vi "Generate_WayPoints_ConstantDistance_Unidirection_DPS_and_CV_V2.vi"(11 "Input Cluster":T2={"Scan Rate (um/s)"=15.0, "X Start"=15.0, "X End"=15.0, "Y Start"=15.0, "Y End"=15.0, "Z Start"=15.0, "Moving Distance (um)"=1.0, "V"=15.0, "Z End"=15.0, "V2"=15.0, "Approach Rate (um/s)"=15.0, "V3"=15.0, "CV Rate (V/s)"=15.0, " V4"=15.0, "V1"=15.0, "Hold Time1 (ms)"=15, "Hold Time2 (ms)"=15, "Hold Time3 (ms)"=15, "Hold Time4 (ms)"=15, "Hold Time5 (ms)"=15, "Update Position Loop Wait Time (us)"=50000, " V5"=15.0, "Hold Time at each point (ms)"=2, "Backward rate (um/s)"=15.0, "Double potential step feedback? (T/F)"=TRUE, "Hold Time6 (ms)"=15, "Hold Time6 (ms) after move"=15, "From V5 to V,\npotential step (true) or\npotential sweep (false)"=TRUE}) -> (0 "output cluster":T1)   [LabVIEW 2023]
uses:
  TypeDefs/WayPointCluster.ctl
panel:
  in  "WayPointCluster":T1
  out "Y  P":dbl
  out "X  P":dbl
  out "HoppingDistanceX":dbl
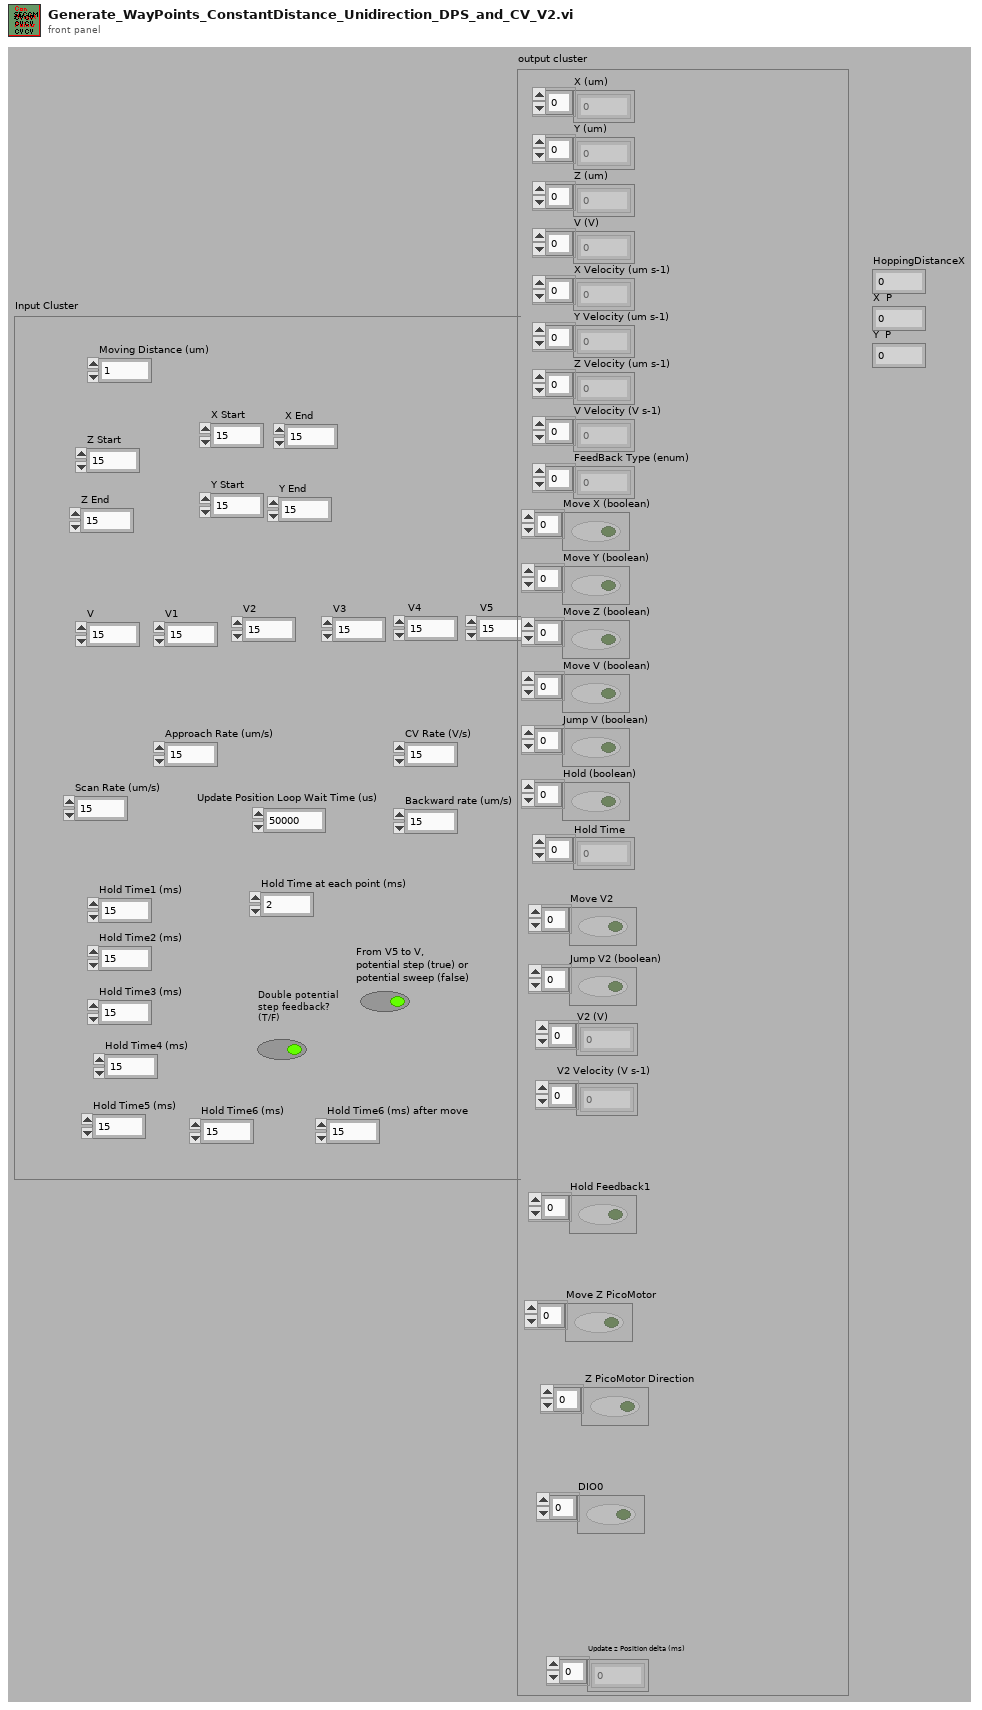
[diagram p1: front panel]
types:
  T1 = typedef "WayPointCluster.ctl" = cluster{"X (um)":dbl[], "Y (um)":dbl[], "Z (um)":dbl[], "V (V)":dbl[], "X Velocity (um s-1)":dbl[], "Y Velocity (um s-1)":dbl[], "Z Velocity (um s-1)":dbl[], "V Velocity (V s-1)":dbl[], "FeedBack Type (enum)":u16[], "Move X (boolean)":bool[], "Move Y (boolean)":bool[], "Move Z (boolean)":bool[], "Move V (boolean)":bool[], "Jump V (boolean)":bool[], "Hold (boolean)":bool[], "Hold Time":u32[], "V2 (V)":dbl[], "Move V2":bool[], "V2 Velocity (V s-1)":dbl[], "Jump V2 (boolean)":bool[], "Update z Position delta (ms)":i16[], "Hold Feedback1":bool[], "Move Z PicoMotor":bool[], " Z PicoMotor Direction":bool[], "DIO0":bool[]}
  T2 = cluster{"Scan Rate (um/s)":dbl, "X Start":dbl, "X End":dbl, "Y Start":dbl, "Y End":dbl, "Z Start":dbl, "Moving Distance (um)":dbl, "V":dbl, "Z End":dbl, "V2":dbl, "Approach Rate (um/s)":dbl, "V3":dbl, "CV Rate (V/s)":dbl, " V4":dbl, "V1":dbl, "Hold Time1 (ms)":i32, "Hold Time2 (ms)":i32, "Hold Time3 (ms)":i32, "Hold Time4 (ms)":i32, "Hold Time5 (ms)":i32, "Update Position Loop Wait Time (us)":u32, " V5":dbl, "Hold Time at each point (ms)":i32, "Backward rate (um/s)":dbl, "Double potential step feedback? (T/F)":bool, "Hold Time6 (ms)":i32, "Hold Time6 (ms) after move":i32, "From V5 to V,\npotential step (true) or\npotential sweep (false)":bool}
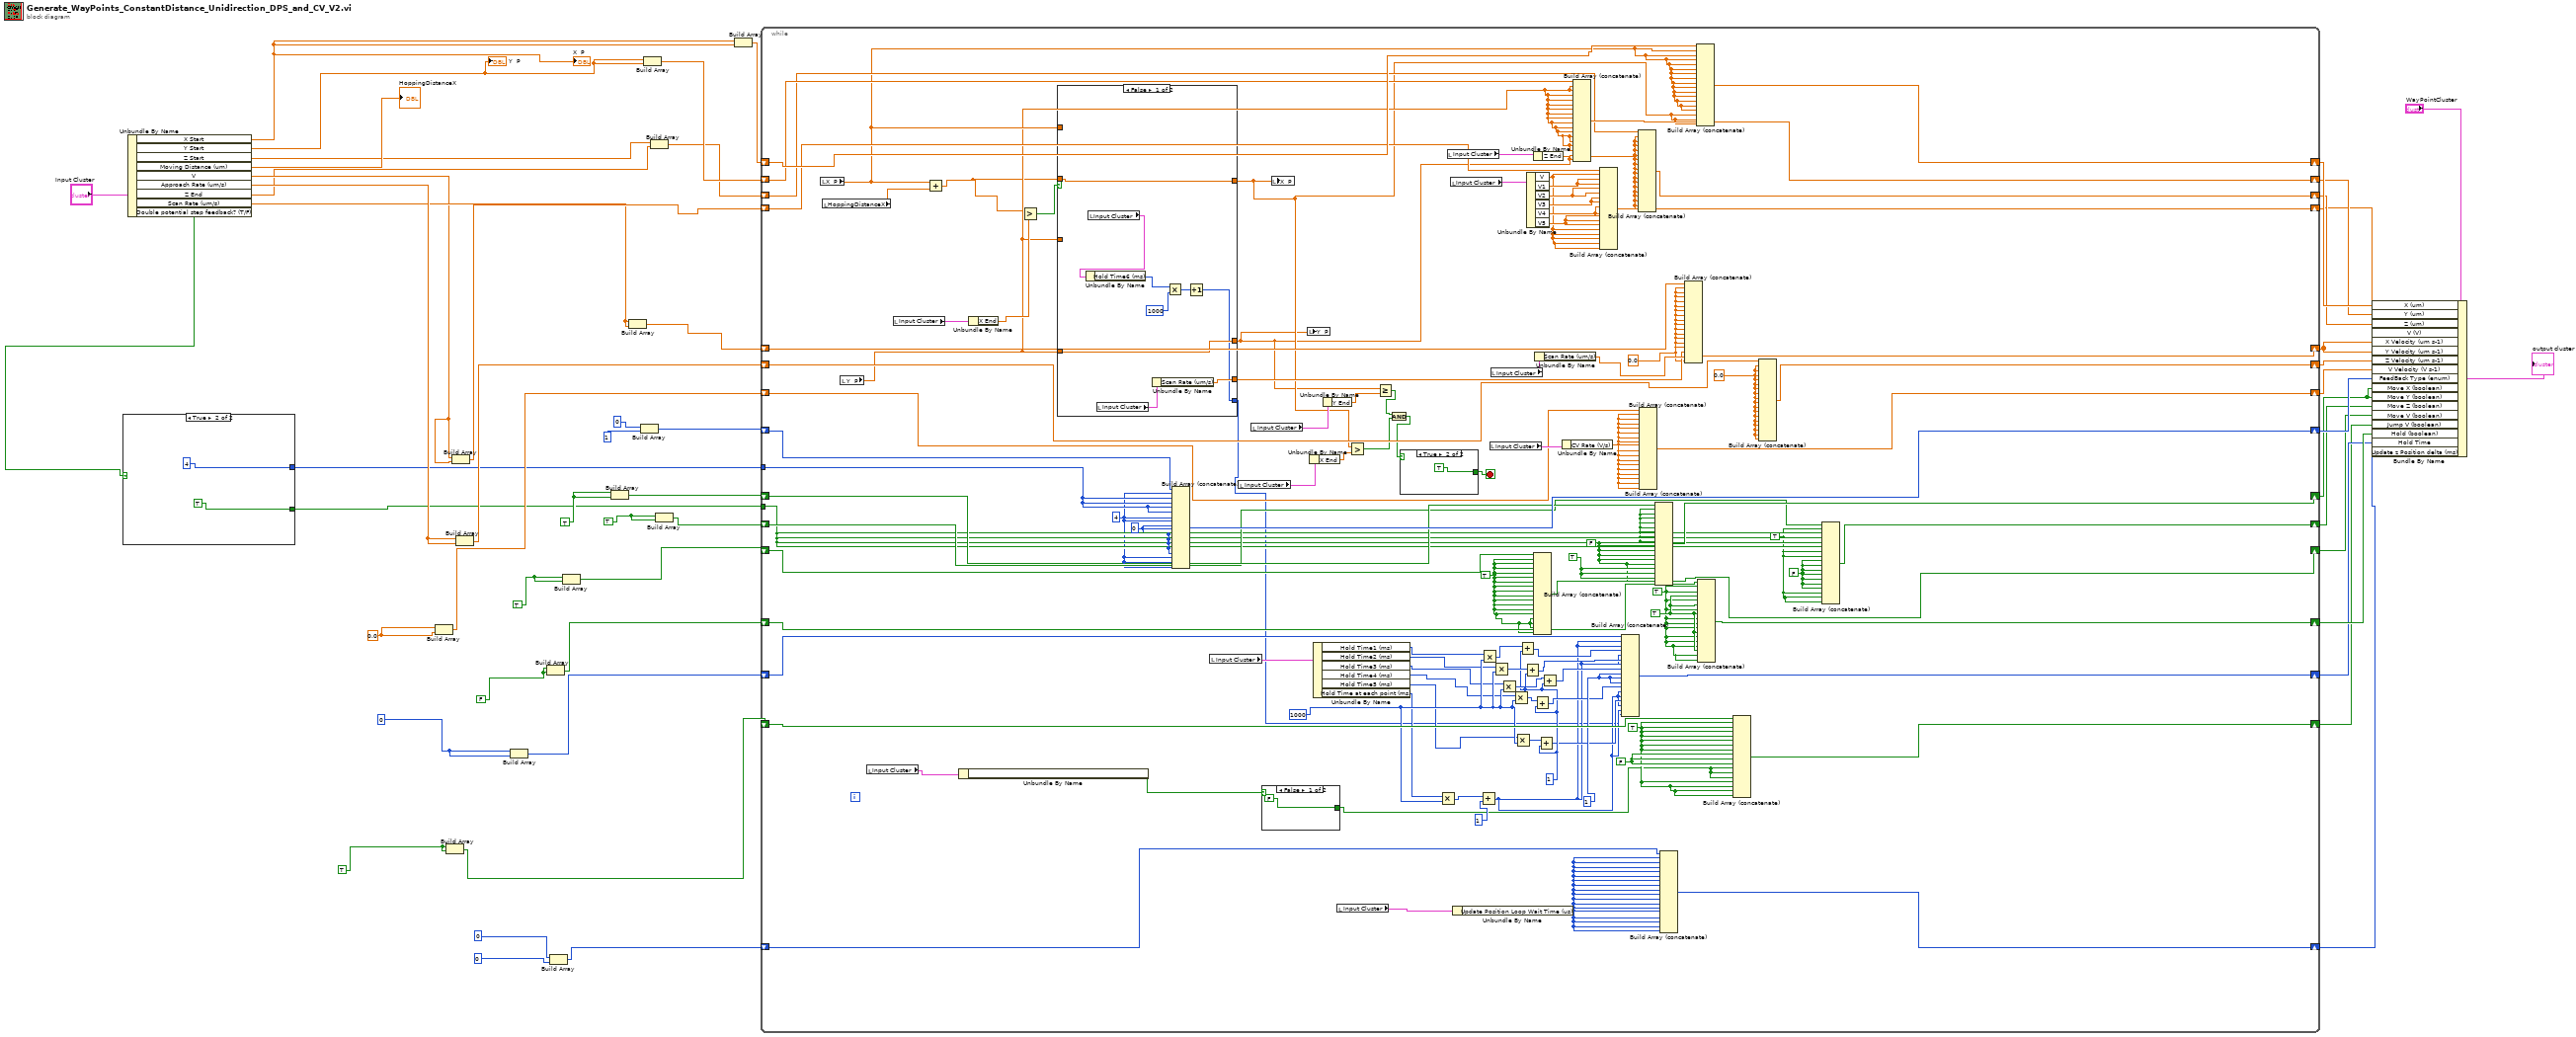
[diagram p0: block diagram]
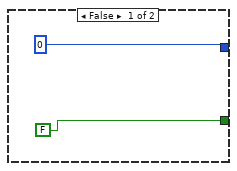
[diagram p2: hidden frame]
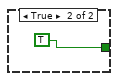
[diagram p3: hidden frame]
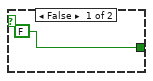
[diagram p4: hidden frame]
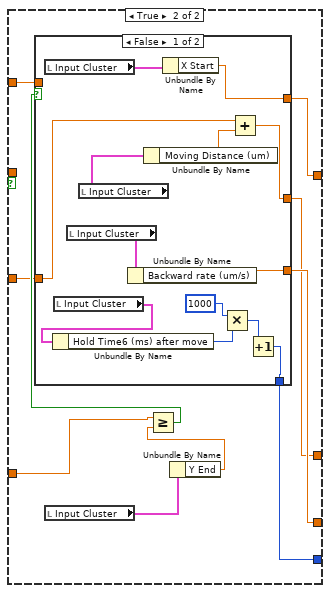
[diagram p5: hidden frame]
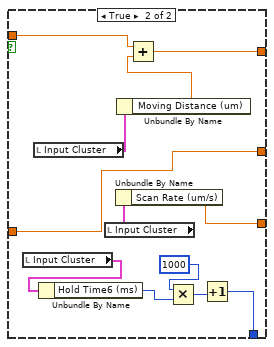
[diagram p6: hidden frame]
diagram:
  w6 = TRUE
  w17 = TRUE
  w18 = u32 0 ("element")
  w15 = FALSE
  w16 = TRUE
  w21 = TRUE
  w19 = 0.0 ("element")
  n1 = Unbundle By Name("Input Cluster") -> ("X Start"=w23:dbl, "Y Start"=w8:dbl, "Z Start"=w34:dbl, "Moving Distance (um)"=→"HoppingDistanceX":dbl, "V"=w20:dbl, "Approach Rate (um/s)"=w27:dbl, "Z End"=w7:dbl, "Scan Rate (um/s)"=w22:dbl, "Double potential step feedback? (T/F)"=w3:bool)
  "X  P" <- w23
  "Y  P" <- w8
  n2 = case shown="True" w3 {
    tunnel: [u16 0 ("element") u16 4 ("element")] -> w2
    tunnel: [FALSE TRUE] -> w1
    frame False {
    }
    frame True {
    }
  }
  n3 = Build Array(w19, w19) -> (w25:dbl[])
  n4 = Build Array(w17, w17) -> (w24:bool[])
  n5 = Build Array(w20, w20) -> (w29:dbl[])
  n6 = Build Array(w27, w27) -> (w26:dbl[])
  n7 = Build Array(w18, w18) -> (w30:u32[])
  n8 = Build Array(w15, w15) -> (w31:bool[])
  n9 = Build Array(u16 0 ("element"), u16 0 ("element")) -> (w12:u16[])
  n10 = Build Array(w21, w21) -> (w32:bool[])
  n11 = Build Array(w16, w16) -> (w33:bool[])
  n12 = Build Array(w22, w22) -> (w28:dbl[])
  n13 = Build Array(u16 0 ("element"), u16 1 ("element")) -> (w47:u16[])
  n14 = Build Array(w8, w8) -> (w36:dbl[])
  n15 = Build Array(w34, w7) -> (w35:dbl[])
  n16 = Build Array(w6, w6) -> (w5:bool[])
  n17 = Build Array(w23, w23) -> (w37:dbl[])
  n18 = while {
    shift-right: [w155] -> w53
    shift-left: w37 -> [w156]
    shift-right: [w153] -> w52
    shift-left: w36 -> [w154]
    shift-right: [w151] -> w51
    shift-left: w35 -> [w152]
    shift-right: [w147] -> w50
    shift-left: w29 -> [w148]
    shift-right: [w149] -> w9
    shift-left: w28 -> [w150]
    shift-right: [w145] -> w49
    shift-left: w26 -> [w146]
    shift-right: [w143] -> w48
    shift-left: w25 -> [w144]
    shift-right: [w162] -> w46
    shift-left: w47 -> [w163]
    shift-right: [w141] -> w44
    shift-left: w33 -> [w142]
    shift-right: [w138] -> w43
    shift-left: w31 -> [w139]
    shift-right: [w136] -> w42
    shift-left: w30 -> [w137]
    shift-right: [w133] -> w41
    shift-left: w24 -> [w134]
    shift-right: [w113] -> w10
    shift-left: w32 -> [w140]
    shift-right: [w131] -> w11
    shift-left: w12 -> [w132]
    shift-right: [w112] -> w4
    shift-left: w5 -> [w111]
    tunnel: w2 -> [w89]
    tunnel: w1 -> [w88]
    stop <- w121 stop-if-true
    w94 = 1 ("element")
    w110 = 1 ("element")
    w78 = FALSE
    w69 = TRUE
    w79 = u16 0 ("element")
    w120 = 1000 ("element")
    w64 = TRUE
    w66 = TRUE
    w122 = FALSE
    w123 = TRUE
    w67 = TRUE
    w68 = FALSE
    w105 = TRUE
    w70 = u16 4 ("element")
    w73 = 0.0 ("element")
    w72 = 0.0 ("element")
    n19 = local read "X  P"() -> (w82:dbl)
    n20 = local read "HoppingDistanceX"() -> (w109:dbl)
    n21 = local read "Y  P"() -> (w81:dbl)
    n22 = local read "Input Cluster"() -> (w62:T2)
    n23 = local read "Input Cluster"() -> (w164:T2)
    n24 = Add(x=w82, y=w109) -> (x+y=w80:dbl)
    n25 = Unbundle By Name(w62) -> ("From V5 to V,\npotential step (true) or\npotential sweep (false)"=w61:bool)
    n26 = Unbundle By Name(w164) -> ("X End"=w159:dbl)
    n27 = Greater?(x=w80, y=w159) -> (0:w107:bool)
    n28 = case shown="False" w107 {
      tunnel: w81 -> [w177 w185]
      tunnel: [w177 w179] -> w76
      tunnel: [w174 w181] -> w77
      tunnel: [w175 w187] -> w104
      tunnel: w82 -> [_ w182]
      tunnel: w81 -> [_ w180]
      tunnel: w80 -> [w174 _]
      tunnel: [w169 w178] -> w63
      frame False {
        n29 = local read "Input Cluster"() -> (w173:T2)
        n30 = Unbundle By Name(w173) -> ("Hold Time6 (ms)"=w172:i32)
        n31 = local read "Input Cluster"() -> (w176:T2)
        n32 = Unbundle By Name(w176) -> ("Scan Rate (um/s)"=w175:dbl)
        n33 = Multiply(x=w172, y=1000 ("element")) -> (x*y=w170:i32)
        n34 = Increment(x=w170) -> (x+1=w169:i32)
      }
      frame True {
        n35 = local read "Input Cluster"() -> (w186:T2)
        n36 = Unbundle By Name(w186) -> ("Y End"=w184:dbl)
        n37 = Greater Or Equal?(x=w185, y=w184) -> (x >= y?=w183:bool)
        n38 = case shown="False" w183 {
          tunnel: [w196 w206] -> w187
          tunnel: w182 -> [_ w211]
          tunnel: [w195 w209] -> w181
          tunnel: [w193 w208] -> w179
          tunnel: w180 -> [w194 w208]
          tunnel: [w188 w201] -> w178
          frame False {
            n39 = local read "Input Cluster"() -> (w199:T2)
            n40 = local read "Input Cluster"() -> (w192:T2)
            n41 = Unbundle By Name(w192) -> ("Hold Time6 (ms) after move"=w190:i32)
            n42 = local read "Input Cluster"() -> (w200:T2)
            n43 = local read "Input Cluster"() -> (w197:T2)
            n44 = Unbundle By Name(w200) -> ("Backward rate (um/s)"=w196:dbl)
            n45 = Unbundle By Name(w197) -> ("Moving Distance (um)"=w198:dbl)
            n46 = Unbundle By Name(w199) -> ("X Start"=w195:dbl)
            n47 = Multiply(x=1000 ("element"), y=w190) -> (x*y=w189:i32)
            n48 = Add(x=w194, y=w198) -> (x+y=w193:dbl)
            n49 = Increment(x=w189) -> (x+1=w188:i32)
          }
          frame True {
            n50 = local read "Input Cluster"() -> (w205:T2)
            n51 = local read "Input Cluster"() -> (w212:T2)
            n52 = Unbundle By Name(w205) -> ("Hold Time6 (ms)"=w204:i32)
            n53 = local read "Input Cluster"() -> (w207:T2)
            n54 = Unbundle By Name(w207) -> ("Scan Rate (um/s)"=w206:dbl)
            n55 = Unbundle By Name(w212) -> ("Moving Distance (um)"=w210:dbl)
            n56 = Add(x=w211, y=w210) -> (x+y=w209:dbl)
            n57 = Multiply(x=1000 ("element"), y=w204) -> (x*y=w202:i32)
            n58 = Increment(x=w202) -> (x+1=w201:i32)
          }
        }
      }
    }
    n59 = Build Array (concatenate)(w163, w70, w89, w89, w89, w89, w70, w70, w79, w79, w79, w79, w79, w79, w79, w70, w70, w70) -> (w162:u16[])
    n60 = local read "Input Cluster"() -> (w135:T2)
    n61 = local read "Input Cluster"() -> (w87:T2)
    n62 = local read "Input Cluster"() -> (w158:T2)
    n63 = case shown="False" w61 {
      tunnel: [FALSE TRUE] -> w60
      frame False {
      }
      frame True {
      }
    }
    n64 = local write "X  P"(w77) -> ()
    n65 = local write "Y  P"(w76) -> ()
    n66 = Unbundle By Name(w87) -> ("X End"=w86:dbl)
    n67 = Unbundle By Name(w135) -> ("Hold Time1 (ms)"=w119:i32, "Hold Time2 (ms)"=w118:i32, "Hold Time3 (ms)"=w117:i32, "Hold Time4 (ms)"=w116:i32, "Hold Time5 (ms)"=w115:i32, "Hold Time at each point (ms)"=w114:i32)
    n68 = Unbundle By Name(w158) -> ("Y End"=w108:dbl)
    n69 = local read "Input Cluster"() -> (w130:T2)
    n70 = Greater?(x=w77, y=w86) -> (0:w84:bool)
    n71 = Greater Or Equal?(x=w76, y=w108) -> (x >= y?=w85:bool)
    n72 = And(x=w85, y=w84) -> (x .and. y?=w83:bool)
    n73 = case shown="True" w83 {
      tunnel: [FALSE TRUE] -> w121
      frame False {
      }
      frame True {
      }
    }
    n74 = Multiply(x=w114, y=w120) -> (x*y=w92:i32)
    n75 = local read "Input Cluster"() -> (w161:T2)
    n76 = local read "Input Cluster"() -> (w160:T2)
    n77 = Unbundle By Name(w130) -> ("Update Position Loop Wait Time (us)"=w65:u32)
    n78 = Add(x=w92, y=1 ("element")) -> (x+y=w90:i32)
    n79 = Multiply(x=w119, y=w120) -> (x*y=w103:i32)
    n80 = local read "Input Cluster"() -> (w157:T2)
    n81 = local read "Input Cluster"() -> (w129:T2)
    n82 = Multiply(x=w118, y=w120) -> (x*y=w101:i32)
    n83 = Multiply(x=w117, y=w120) -> (x*y=w99:i32)
    n84 = Multiply(x=w116, y=w120) -> (x*y=w97:i32)
    n85 = Multiply(x=w115, y=w120) -> (x*y=w95:i32)
    n86 = Add(x=w103, y=w94) -> (x+y=w102:i32)
    n87 = Add(x=w101, y=w94) -> (x+y=w100:i32)
    n88 = Unbundle By Name(w160) -> ("V"=w75:dbl, "V1"=w128:dbl, "V2"=w127:dbl, "V3"=w126:dbl, "V4"=w125:dbl, "V5"=w124:dbl)
    n89 = Unbundle By Name(w161) -> ("Z End"=w74:dbl)
    n90 = Build Array (concatenate)(w140, w66, w66, w66, w66, w66, w66, w66, w66, w66, w66, w66, w66, w66, w66, w66, w66, w66) -> (w113:bool[])
    n91 = Add(x=w97, y=w94) -> (x+y=w96:i32)
    n92 = Unbundle By Name(w129) -> ("Scan Rate (um/s)"=w106:dbl)
    n93 = Add(x=w95, y=w94) -> (x+y=w93:i32)
    n94 = Add(x=w99, y=w94) -> (x+y=w98:i32)
    n95 = Unbundle By Name(w157) -> ("CV Rate (V/s)"=w71:dbl)
    n96 = Build Array (concatenate)(w154, w81, w81, w81, w81, w81, w81, w81, w81, w81, w81, w81, w81, w81, w81, w81, w76, w76) -> (w153:dbl[])
    n97 = Build Array (concatenate)(w148, w75, w128, w128, w127, w127, w126, w126, w125, w125, w124, w124, w124, w75, w75, w75, w75, w75) -> (w147:dbl[])
    n98 = Build Array (concatenate)(w137, w90, w90, w102, w90, w100, w90, w98, w110, w110, w110, w96, w90, w90, w93, w90, w90, w63) -> (w136:u32[])
    n99 = Build Array (concatenate)(w152, w74, w74, w74, w74, w74, w74, w74, w74, w74, w74, w74, w74, w74, w74, w74, w74, w74) -> (w151:dbl[])
    n100 = Build Array (concatenate)(w144, w71, w71, w71, w71, w71, w71, w71, w71, w71, w71, w71, w71, w71, w71, w71, w71, w71) -> (w143:dbl[])
    n101 = Build Array (concatenate)(w142, w68, w68, w68, w68, w68, w68, w68, w68, w68, w68, w68, w68, w68, w105, w105, w105, w68) -> (w141:bool[])
    n102 = Build Array (concatenate)(w132, w65, w65, w65, w65, w65, w65, w65, w65, w65, w65, w65, w65, w65, w65, w65, w65, w65) -> (w131:u32[])
    n103 = Build Array (concatenate)(w150, w73, w73, w73, w73, w73, w73, w73, w73, w73, w73, w73, w73, w73, w73, w104, w106, w73) -> (w149:dbl[])
    n104 = Build Array (concatenate)(w156, w82, w82, w82, w82, w82, w82, w82, w82, w82, w82, w82, w82, w82, w82, w77, w77, w77) -> (w155:dbl[])
    n105 = Build Array (concatenate)(w139, w67, w67, w123, w67, w123, w67, w123, w67, w67, w67, w123, w67, w67, w67, w123, w67, w67) -> (w138:bool[])
    n106 = Build Array (concatenate)(w134, w64, w64, w64, w64, w64, w64, w64, w122, w122, w122, w60, w60, w60, w64, w64, w64, w64) -> (w133:bool[])
    n107 = Build Array (concatenate)(w146, w72, w72, w72, w72, w72, w72, w72, w72, w72, w72, w72, w72, w72, w72, w72, w72, w72) -> (w145:dbl[])
    n108 = Build Array (concatenate)(w111, w69, w88, w88, w88, w88, w69, w69, w78, w78, w78, w78, w78, w78, w78, w69, w69, w69) -> (w112:bool[])
  }
  n109 = Bundle By Name(cluster="WayPointCluster", "X (um)"=w53, "Y (um)"=w52, "Z (um)"=w51, "V (V)"=w50, "X Velocity (um s-1)"=w9, "Y Velocity (um s-1)"=w9, "Z Velocity (um s-1)"=w49, "V Velocity (V s-1)"=w48, "FeedBack Type (enum)"=w46, "Move X (boolean)"=w44, "Move Y (boolean)"=w44, "Move Z (boolean)"=w4, "Move V (boolean)"=w10, "Jump V (boolean)"=w41, "Hold (boolean)"=w43, "Hold Time"=w42, "Update z Position delta (ms)"=w11) -> (→"output cluster":T1)
